vi "RGB LED Write.vi"(0 "Arduino Resource":T1={"VISA resource"="", "Board Type"=enum."Uno", "Connection Type"=enum."USB / Serial", "Bytes Per Packet (15)"=15}, 5 "RGB LED Pins":u8[](array[numeric]), 9 "Color":u32(colorbox), 11 "error in":errorcluster) -> (4 "Arduino Resource":T1={"VISA resource"="", "Board Type"=enum."Uno", "Connection Type"=enum."USB / Serial", "Bytes Per Packet (15)"=15}, 8 "RGB LED Pins Out":u8[](array[numeric]), 15 "error out":errorcluster)   [LabVIEW 2011, in "LabVIEW Interface for Arduino.lvlib"]
doc: "Write color value to RGB LED. Arduino Configure RGB LED must be called to configure the RGB LED pins before calling this VI."
uses:
  <vilib>/LabVIEW Interface for Arduino/LabVIEW Interface for Arduino.lvlib
  <vilib>/LabVIEW Interface for Arduino/Private/Type Defs/Arduino Resource.ctl
  <vilib>/LabVIEW Interface for Arduino/Private/Type Defs/Board Type.ctl
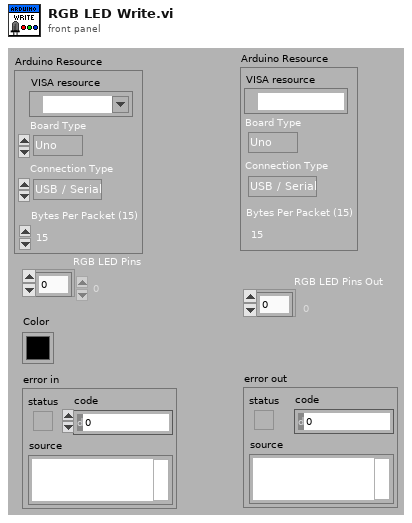
[diagram p1: front panel]
types:
  T1 = typedef "LabVIEW Interface for Arduino.lvlib/Arduino Resource.ctl" = cluster{"VISA resource":refnum<visa-resource-name>, "Board Type":T2, "Connection Type":enum8{"USB / Serial"}, "Bytes Per Packet (15)":u8}
  T2 = typedef "LabVIEW Interface for Arduino.lvlib/Board Type.ctl" = enum16{"Uno", "Dimuelanove w/Atmega 328", "Mega 2560"}
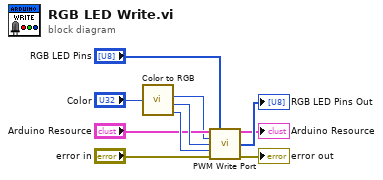
[diagram p0: block diagram]
diagram:
  n1 = call <vilib>:"Color to RGB.vi"("Color"="Color") -> ("R"=w1:u8, "G"=w8:u8, "B"=w7:u8)  [unwired: 1 out]
  n2 = call <vilib>:"PWM Write Port.vi"("Arduino Resource"="Arduino Resource", "PWM Pins"="RGB LED Pins", "PWM 0 (0-255)"=w1, "PWM 1 (0-255)"=w8, "PWM 2 (0-255)"=w7, "error in"="error in") -> ("Arduino Resource"=→"Arduino Resource":T1, "PWM Pins"=→"RGB LED Pins Out":u8[], "error out"=→"error out":errorcluster)  [unwired: 7 in]
